vi "Stat2Double.vi"(10 "Numeric in":u32, 11 "Stat Address":T1 items=["Torque Enable", "Homing Complete", "Goal Id", "Goal Iq", "Goal Velo", "Goal Posi", "Present Id", "Present Iq", "Present Velo", "Present Posi", "Bus Voltage", "Temperature Winding", "Temperature MOSFET", "Temperature IC", "Error Status", "Iq_Temps"]) -> (3 "Numeric out":dbl)   [LabVIEW 2016, in "GEN_2.lvlib"]
uses:
  GEN_2.lvlib
  GEN2_Stat_Addr.ctl
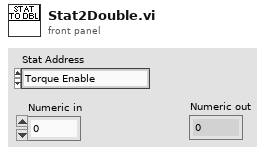
[diagram p1: front panel]
types:
  T1 = typedef "GEN_2.lvlib/GEN2_Stat_Addr.ctl" = u8
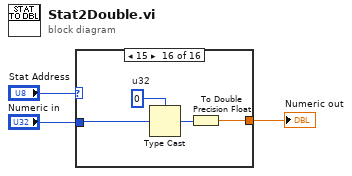
[diagram p0: block diagram]
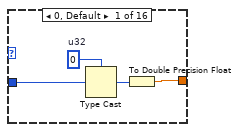
[diagram p2: hidden frame]
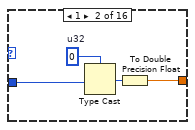
[diagram p3: hidden frame]
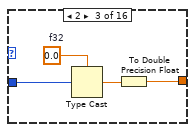
[diagram p4: hidden frame]
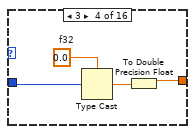
[diagram p5: hidden frame]
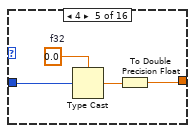
[diagram p6: hidden frame]
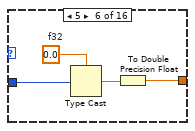
[diagram p7: hidden frame]
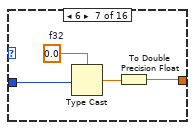
[diagram p8: hidden frame]
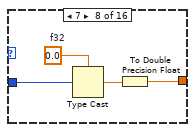
[diagram p9: hidden frame]
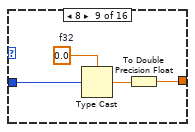
[diagram p10: hidden frame]
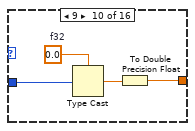
[diagram p11: hidden frame]
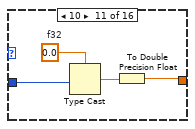
[diagram p12: hidden frame]
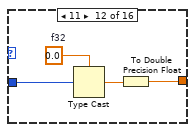
[diagram p13: hidden frame]
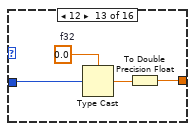
[diagram p14: hidden frame]
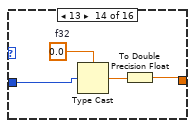
[diagram p15: hidden frame]
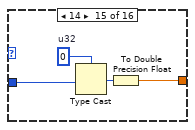
[diagram p16: hidden frame]
diagram:
  n1 = case shown="15" "Stat Address" {
    tunnel: "Numeric in" -> [w6 w9 w13 w16 w21 w25 w29 w33 w37 w41 w45 w49 w52 w56 w60 w65]
    tunnel: [w4 w8 w12 w17 w20 w24 w28 w32 w36 w40 w44 w48 w53 w57 w61 w64] -> w3
    frame 0, Default {
      w7 = u32 0  # u32
      n2 = Type Cast(type=w7, x=w6) -> (*(type *) &x=w5:u32)
      n3 = To Double Precision Float(number=w5) -> (double precision float=w4:dbl)
    }
    frame 1 {
      w10 = u32 0  # u32
      n4 = Type Cast(type=w10, x=w9) -> (*(type *) &x=w11:u32)
      n5 = To Double Precision Float(number=w11) -> (double precision float=w8:dbl)
    }
    frame 2 {
      w14 = sgl 0.0  # f32
      n6 = Type Cast(type=w14, x=w13) -> (*(type *) &x=w15:sgl)
      n7 = To Double Precision Float(number=w15) -> (double precision float=w12:dbl)
    }
    frame 3 {
      w19 = sgl 0.0  # f32
      n8 = Type Cast(type=w19, x=w16) -> (*(type *) &x=w18:sgl)
      n9 = To Double Precision Float(number=w18) -> (double precision float=w17:dbl)
    }
    frame 4 {
      w23 = sgl 0.0  # f32
      n10 = Type Cast(type=w23, x=w21) -> (*(type *) &x=w22:sgl)
      n11 = To Double Precision Float(number=w22) -> (double precision float=w20:dbl)
    }
    frame 5 {
      w27 = sgl 0.0  # f32
      n12 = Type Cast(type=w27, x=w25) -> (*(type *) &x=w26:sgl)
      n13 = To Double Precision Float(number=w26) -> (double precision float=w24:dbl)
    }
    frame 6 {
      w31 = sgl 0.0  # f32
      n14 = Type Cast(type=w31, x=w29) -> (*(type *) &x=w30:sgl)
      n15 = To Double Precision Float(number=w30) -> (double precision float=w28:dbl)
    }
    frame 7 {
      w35 = sgl 0.0  # f32
      n16 = Type Cast(type=w35, x=w33) -> (*(type *) &x=w34:sgl)
      n17 = To Double Precision Float(number=w34) -> (double precision float=w32:dbl)
    }
    frame 8 {
      w39 = sgl 0.0  # f32
      n18 = Type Cast(type=w39, x=w37) -> (*(type *) &x=w38:sgl)
      n19 = To Double Precision Float(number=w38) -> (double precision float=w36:dbl)
    }
    frame 9 {
      w43 = sgl 0.0  # f32
      n20 = Type Cast(type=w43, x=w41) -> (*(type *) &x=w42:sgl)
      n21 = To Double Precision Float(number=w42) -> (double precision float=w40:dbl)
    }
    frame 10 {
      w46 = sgl 0.0  # f32
      n22 = Type Cast(type=w46, x=w45) -> (*(type *) &x=w47:sgl)
      n23 = To Double Precision Float(number=w47) -> (double precision float=w44:dbl)
    }
    frame 11 {
      w51 = sgl 0.0  # f32
      n24 = Type Cast(type=w51, x=w49) -> (*(type *) &x=w50:sgl)
      n25 = To Double Precision Float(number=w50) -> (double precision float=w48:dbl)
    }
    frame 12 {
      w55 = sgl 0.0  # f32
      n26 = Type Cast(type=w55, x=w52) -> (*(type *) &x=w54:sgl)
      n27 = To Double Precision Float(number=w54) -> (double precision float=w53:dbl)
    }
    frame 13 {
      w59 = sgl 0.0  # f32
      n28 = Type Cast(type=w59, x=w56) -> (*(type *) &x=w58:sgl)
      n29 = To Double Precision Float(number=w58) -> (double precision float=w57:dbl)
    }
    frame 14 {
      w62 = u32 0  # u32
      n30 = Type Cast(type=w62, x=w60) -> (*(type *) &x=w63:u32)
      n31 = To Double Precision Float(number=w63) -> (double precision float=w61:dbl)
    }
    frame 15 {
      w67 = u32 0  # u32
      n32 = Type Cast(type=w67, x=w65) -> (*(type *) &x=w66:u32)
      n33 = To Double Precision Float(number=w66) -> (double precision float=w64:dbl)
    }
  }
  "Numeric out" <- w3
